vi "Inputs.vi"() -> ()   [LabVIEW 2017]
panel:
  in  "Act_Vp":dbl
  in  "Act_Vy":dbl
  in  "Act_Vx":dbl
  in  "Stop":bool
  in  "C1/Encoder":i32
  in  "C0/Encoder":i32
  in  "B/Encoder":i32
  in  "A/Encoder":i32
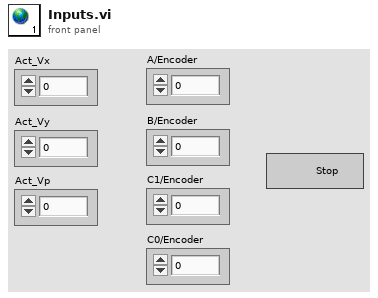
[diagram p1: front panel]
diagram:
